vi "Write_mzMLFile.vi"(8 "error in (no error)":errorcluster, 10 "Signal Segment":T1={"SampleRate"=-1.0, "TrigDelay"=0.0, "SpecLength"=0.0, "DAQ_Range"=0.0, "Average#"=0, "Position"=[], "Spectrum"=[], "Calibr."=[], "Pressure"=-1.0, "Desp_LaserEnergy"=-1.0, "PI_LaserEnergy"=-1.0, "Voltages Table"=[], "ProcMode"=enum."None", "Threshold"=-1.0, "Comment"="", "TickCount"=0.0, "Time Stamp"=timestamp(0 s since 1904-01-01)} {"TickCount" format="%#.2f"}, 11 "Filename":path) -> (0 "error out":errorcluster)   [LabVIEW 2013]
uses:
  Signal_Segment.ctl
  ControlDef/ProcessingMode.ctl
panel:
  out "Sample Rate":dbl=100000000.0
  out "Depth":dbl=16384.0
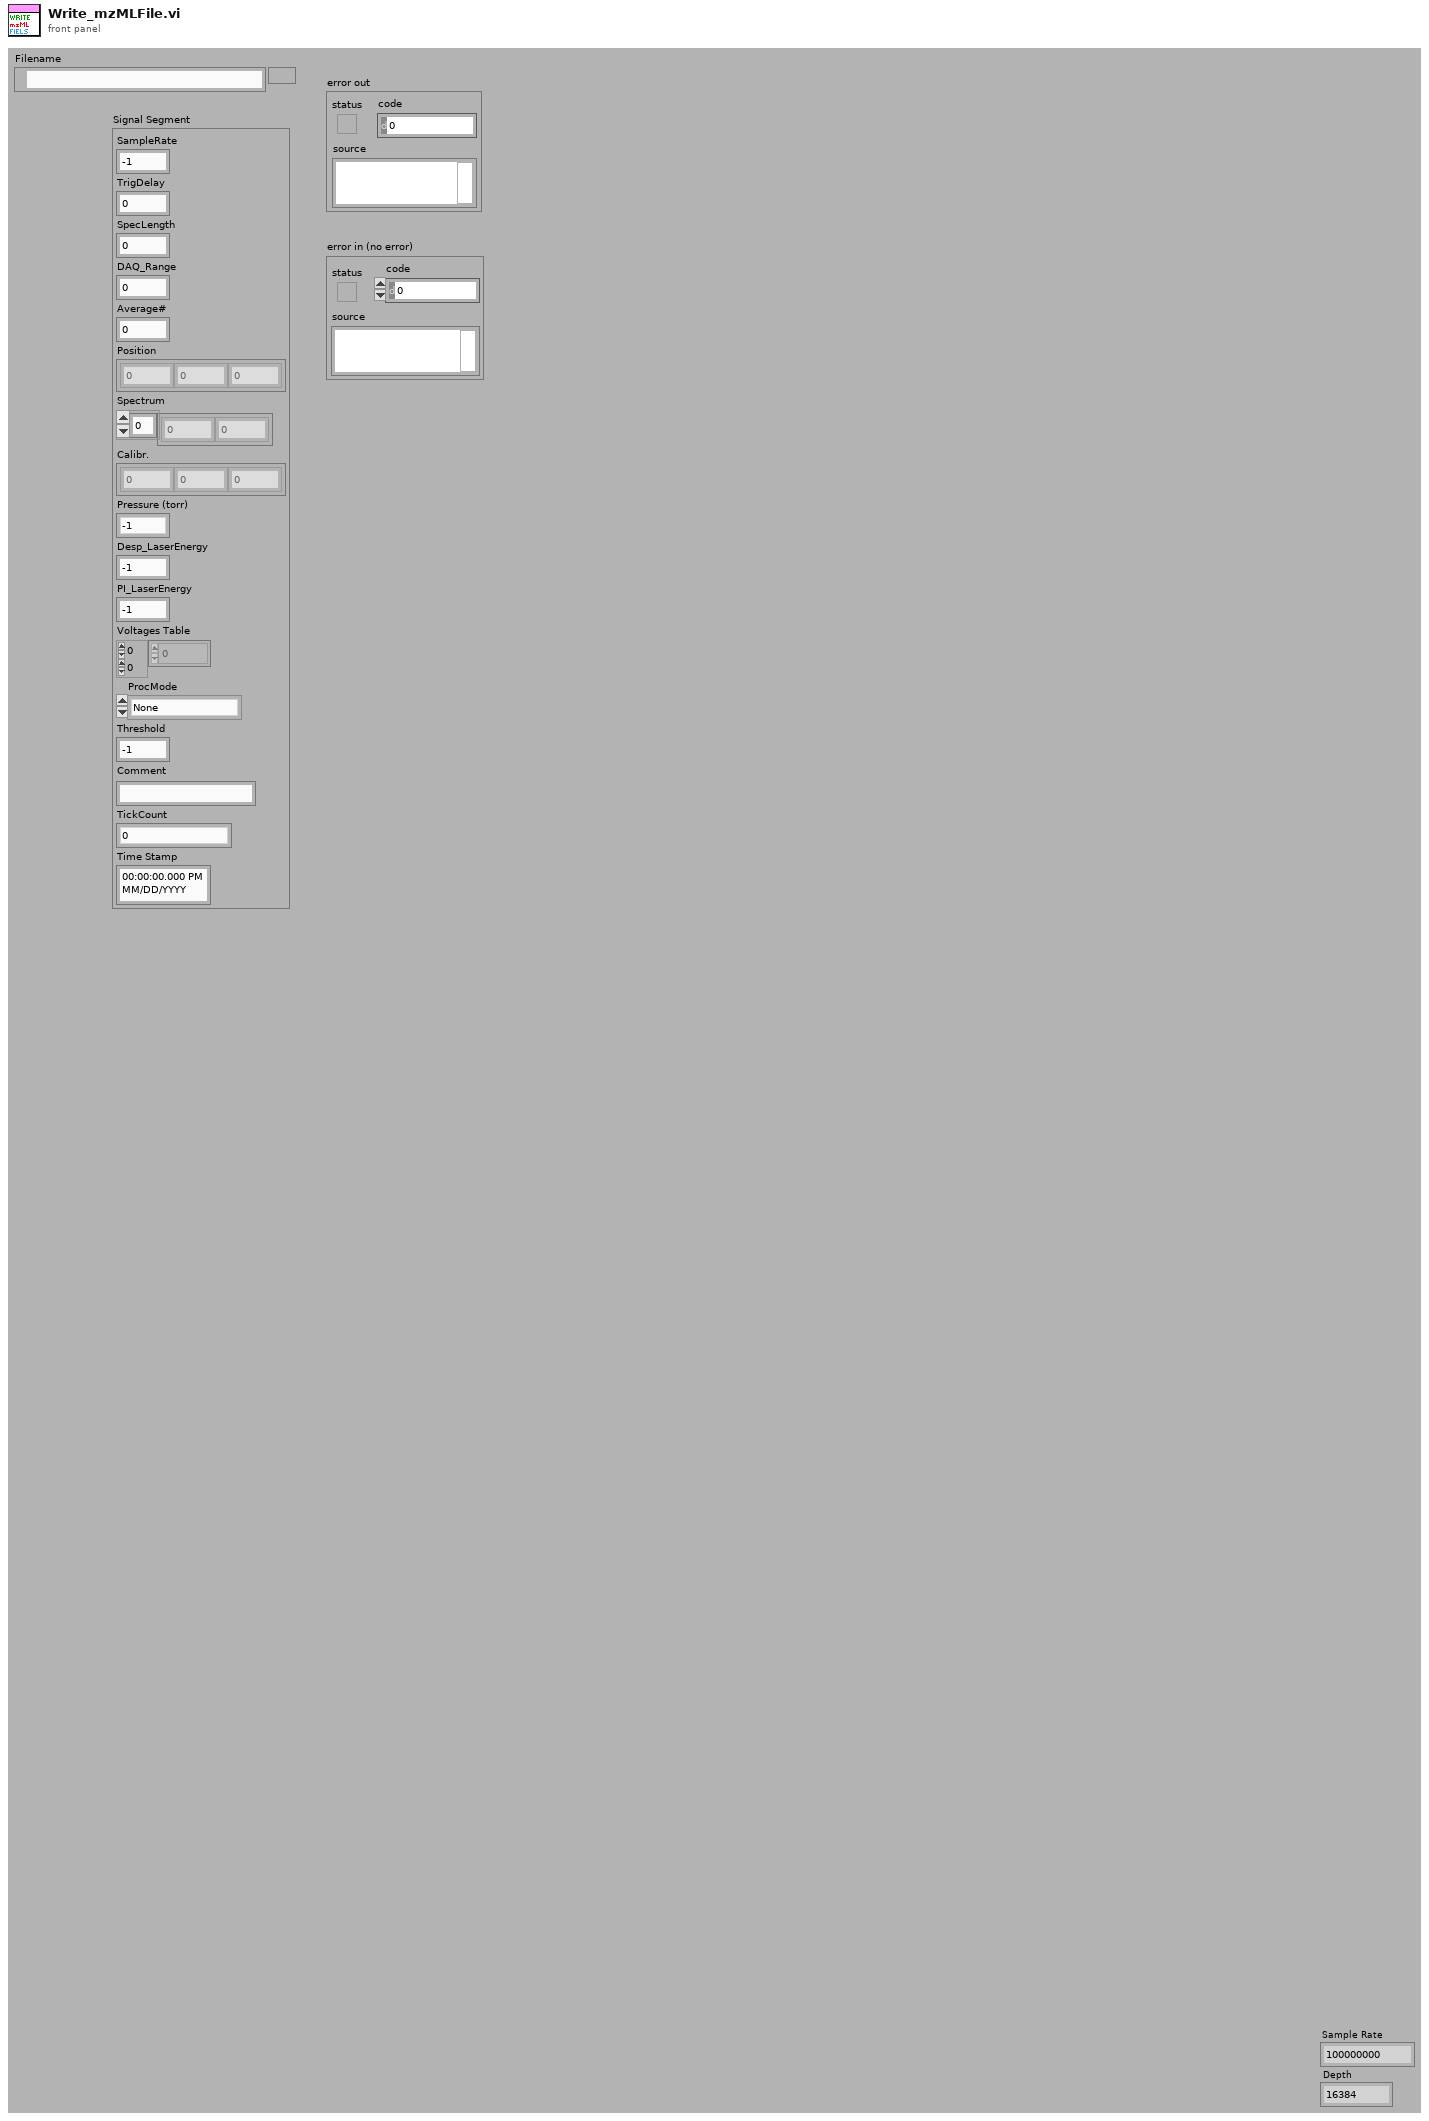
[diagram p1: front panel]
types:
  T1 = typedef "Signal_Segment.ctl" = cluster{"SampleRate":dbl, "TrigDelay":dbl, "SpecLength":dbl, "DAQ_Range":dbl, "Average#":i32, "Position":dbl[], "Spectrum":sgl[], "Calibr.":dbl[], "Pressure":dbl, "Desp_LaserEnergy":dbl, "PI_LaserEnergy":dbl, "Voltages Table":sgl[][], "ProcMode":T2, "Threshold":dbl, "Comment":string, "TickCount":dbl, "Time Stamp":timestamp}
  T2 = typedef "ProcessingMode.ctl" = enum16{"None", "Drop by Threshold", "TDC Simulate", "SetFilter"}
  T3 = enum16{"open", "replace", "create", "open or create", "replace or create", "replace or create with confirmation"}
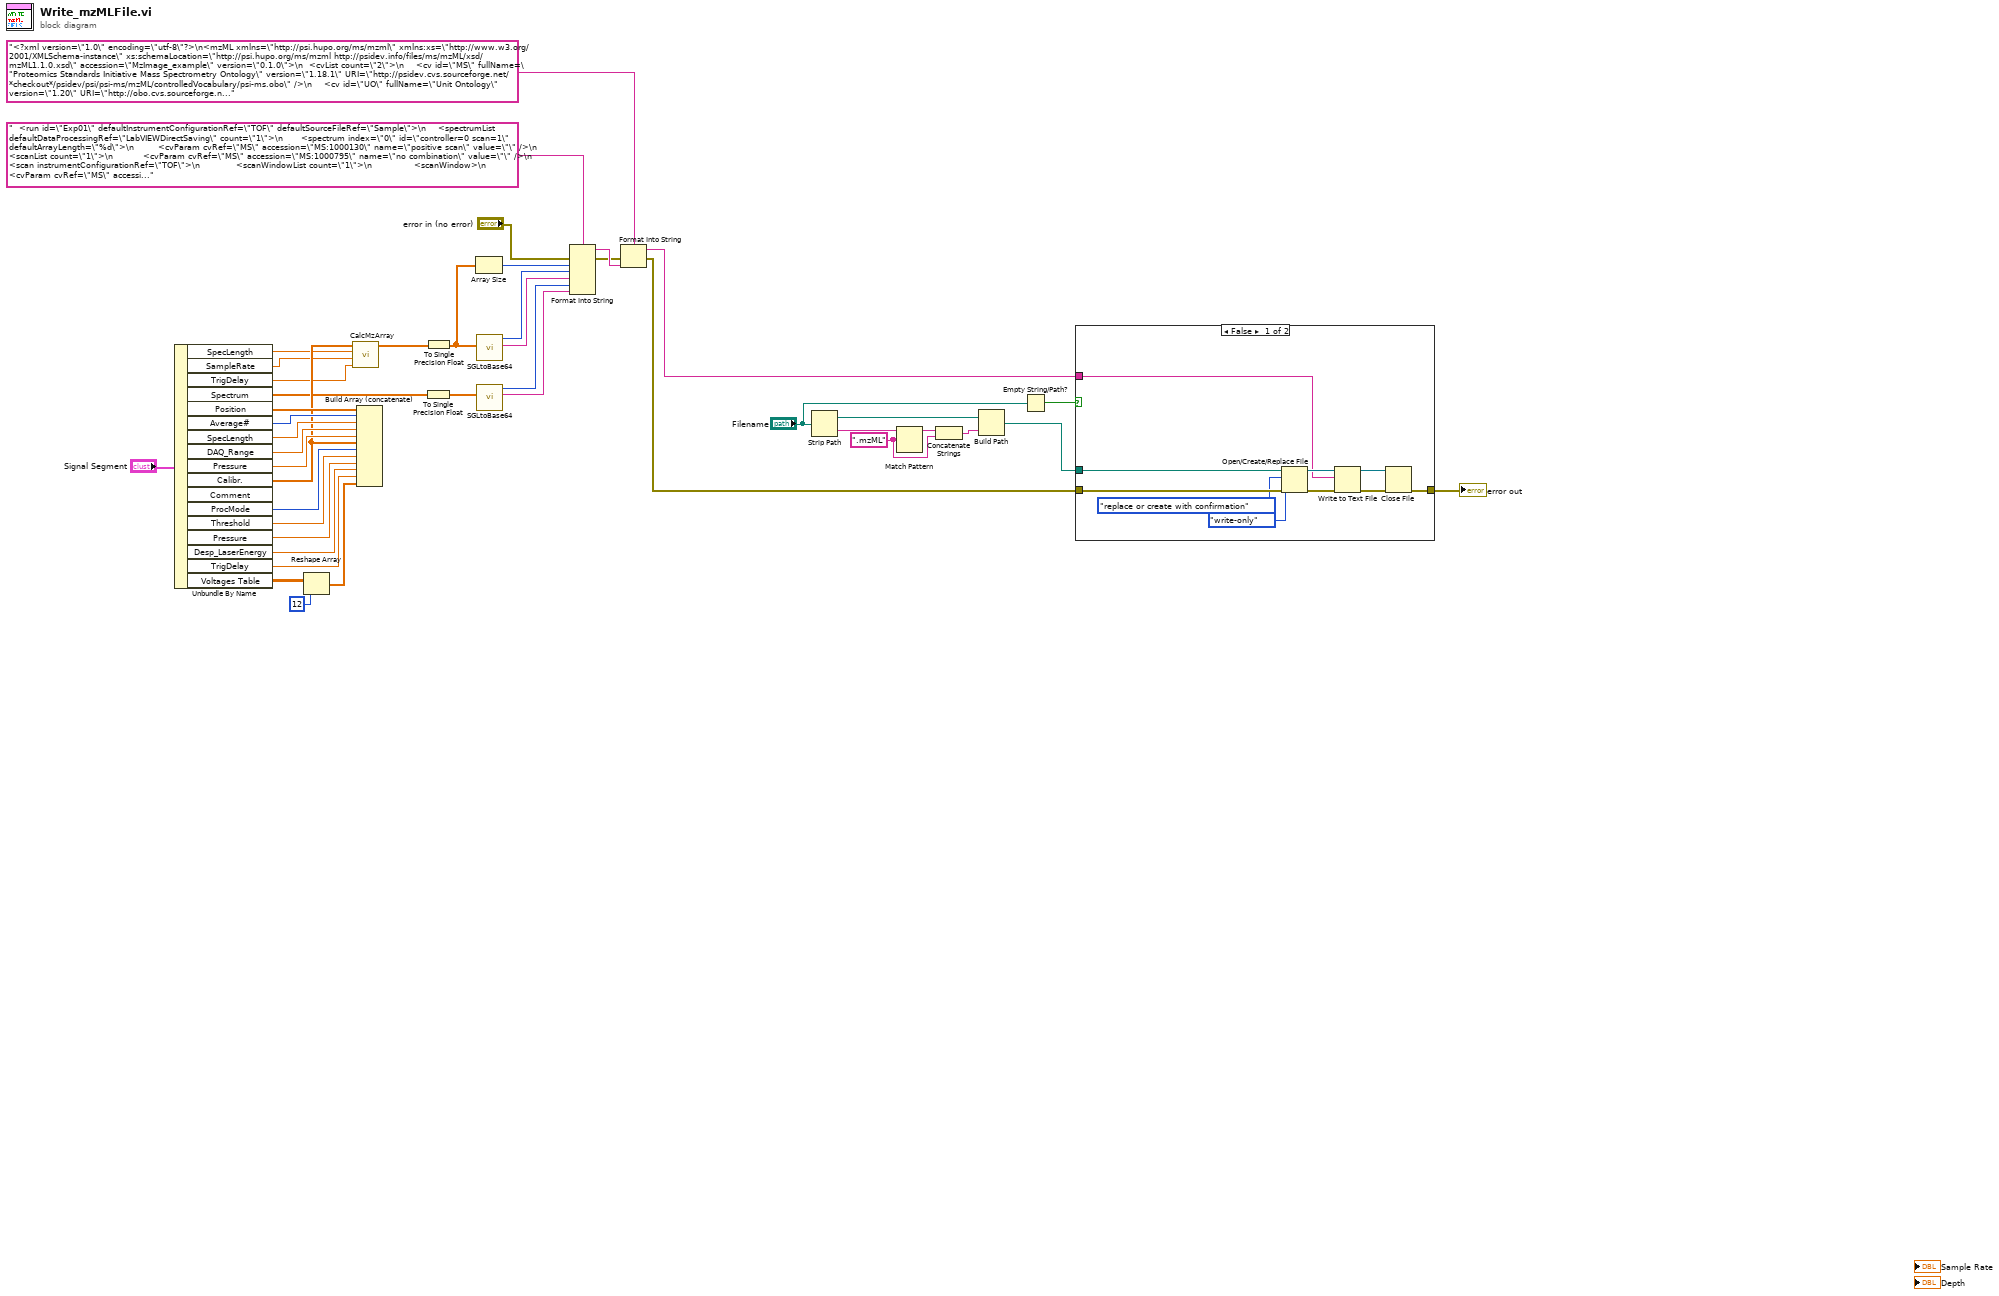
[diagram p0: block diagram]
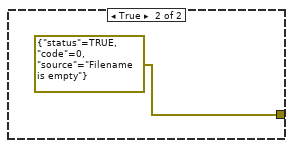
[diagram p2: hidden frame]
diagram:
  w30 = ".mzML" ("regular expression")
  n1 = Unbundle By Name("Signal Segment") -> ("SpecLength"=w2:dbl, "SampleRate"=w1:dbl, "TrigDelay"=w3:dbl, "Spectrum"=w4:sgl[], "Position"=w40:dbl[], "Average#"=w41:i32, "SpecLength"=w38:dbl, "DAQ_Range"=w42:dbl, "Pressure"=w37:dbl, "Calibr."=w21:dbl[], "ProcMode"=w36:T2, "Threshold"=w35:dbl, "Pressure"=w29:dbl, "Desp_LaserEnergy"=w28:dbl, "TrigDelay"=w22:dbl, "Voltages Table"=w24:sgl[][])  [unwired: 1 out]
  n2 = Reshape Array(w24, 12 ("dimension size")) -> (w23:sgl[])
  n3 = call "CalcMzArray.vi"("TrigDelay"=w3, "Sample Rate"=w1, "Depth"=w2, "mzCali. (a/b/c)"=w21) -> ("mzArray"=w5:dbl[])  [unwired: 7 in]
  n4 = Build Array (concatenate)(w40, w41, w38, w42, w37, w21, w36, w35, w29, w28, w22, w23) -> ()  [unwired: 1 out]
  n5 = To Single Precision Float(number=w4) -> (single precision float=w6:sgl[])
  n6 = To Single Precision Float(number=w5) -> (single precision float=w12:sgl[])
  n7 = Array Size(array=w12) -> (size(s)=w11:i32)
  n8 = call "SGLtoBase64.vi"("SGL Array"=w12) -> ("Base64 String"=w16:string, "length"=w15:i32)  [unwired: 9 in]
  n9 = call "SGLtoBase64.vi"("SGL Array"=w6) -> ("Base64 String"=w13:string, "length"=w14:i32)  [unwired: 9 in]
  n10 = Format Into String(format string="  <run id=\"Exp01\" defaultInstrumentConfigurationRef=\"TOF\" defaultSourceFileRef=\"Sample\">\n    <spectrumList defaultDataProcessingRef=\"LabVIEWDirectSaving\" count=\"1\">\n      <spectrum index=\"0\" id=\"controller=0 scan=1\" defaultArrayLength=\"%d\">\n        <cvParam cvRef=\"MS\" accession=\"MS:1000130\" name=\"positive scan\" value=\"\" />\n        <scanList count=\"1\">\n          <cvParam cvRef=\"MS\" accession=\"MS:1000795\" name=\"no combination\" value=\"\" />\n          <scan instrumentConfigurationRef=\"TOF\">\n            <scanWindowList count=\"1\">\n              <scanWindow>\n                <cvParam cvRef=\"MS\" accession=\"MS:1000501\" name=\"scan window lower limit\" value=\"0\" unitCvRef=\"MS\" unitAccession=\"MS:1000040\" unitName=\"m/z\" />\n                <cvParam cvRef=\"MS\" accession=\"MS:1000500\" name=\"scan window upper limit\" value=\"5000\" unitCvRef=\"MS\" unitAccession=\"MS:1000040\" unitName=\"m/z\" />\n              </scanWindow>\n            </scanWindowList>\n          </scan>\n        </scanList>\n        <binaryDataArrayList count=\"2\">\n          <binaryDataArray encodedLength=\"%d\">\n            <cvParam cvRef=\"MS\" accession=\"MS:1000514\" name=\"m/z array\" unitCvRef=\"MS\" unitAccession=\"MS:1000040\" unitName=\"m/z\" />\n            <cvParam cvRef=\"MS\" accession=\"MS:1000576\" name=\"no compression\" />\n            <cvParam cvRef=\"MS\" accession=\"MS:1000521\" name=\"32-bit float\" />\n            <binary>%s</binary>\n          </binaryDataArray>\n          <binaryDataArray encodedLength=\"%d\">\n            <cvParam cvRef=\"MS\" accession=\"MS:1000515\" name=\"intensity array\" unitCvRef=\"MS\" unitAccession=\"MS:1000131\" unitName=\"number of counts\" />\n            <cvParam cvRef=\"MS\" accession=\"MS:1000574\" name=\"zlib compression\" />\n            <cvParam cvRef=\"MS\" accession=\"MS:1000521\" name=\"32-bit float\" />\n            <binary>%s</binary>\n          </binaryDataArray>\n        </binaryDataArrayList>\n      </spectrum>\n    </spectrumList>\n  </run>", error in="error in (no error)", w11, w15, w16, w14, w13) -> (resulting string=w17:string, error out=w9:errorcluster)  [unwired: 1 in]
  n11 = Format Into String(format string="<?xml version=\"1.0\" encoding=\"utf-8\"?>\n<mzML xmlns=\"http://psi.hupo.org/ms/mzml\" xmlns:xs=\"http://www.w3.org/2001/XMLSchema-instance\" xs:schemaLocation=\"http://psi.hupo.org/ms/mzml http://psidev.info/files/ms/mzML/xsd/mzML1.1.0.xsd\" accession=\"MzImage_example\" version=\"0.1.0\">\n  <cvList count=\"2\">\n    <cv id=\"MS\" fullName=\"Proteomics Standards Initiative Mass Spectrometry Ontology\" version=\"1.18.1\" URI=\"http://psidev.cvs.sourceforge.net/*checkout*/psidev/psi/psi-ms/mzML/controlledVocabulary/psi-ms.obo\" />\n    <cv id=\"UO\" fullName=\"Unit Ontology\" version=\"1.20\" URI=\"http://obo.cvs.sourceforge.net/*checkout*/obo/obo/ontology/phenotype/unit.obo\" />\n  </cvList>\n  <fileDescription>\n    <fileContent>\n      <cvParam cvRef=\"MS\" accession=\"MS:1000442\" name=\"spectrum\" />\n    </fileContent>\n    <sourceFileList count=\"2\">\n      <sourceFile id=\"Sample\" name=\"\" location=\"\"></sourceFile>\n    </sourceFileList>\n  </fileDescription>\n  <softwareList count=\"1\">\n    <software id=\"software\" version=\"3.5\">\n      <cvParam cvRef=\"MS\" accession=\"MS:1000531\" name=\"software\" value=\"\" />\n    </software>\n  </softwareList>\n  <instrumentConfigurationList count=\"1\">\n    <instrumentConfiguration id=\"TOF\">\n      <cvParam cvRef=\"MS\" accession=\"MS:1000287\" name=\"time-of-flight mass spectrometer\" value=\"\" />\n      <componentList count=\"3\">\n        <source order=\"1\">\n          <cvParam cvRef=\"MS\" accession=\"MS:1000393\" name=\"laser desorption ionization\"></cvParam>\n        </source>\n        <analyzer order=\"2\">\n          <cvParam cvRef=\"MS\" accession=\"MS:1000084\" name=\"TOF\" value=\"\" />\n        </analyzer>\n        <detector order=\"3\">\n          <cvParam cvRef=\"MS\" accession=\"MS:1000114\" name=\"microchannel plate detector\" value=\"\" />\n        </detector>\n      </componentList>\n      <softwareRef ref=\"software\" />\n    </instrumentConfiguration>\n  </instrumentConfigurationList>\n  <dataProcessingList count=\"1\">\n    <dataProcessing id=\"LabVIEWDirectSaving\">\n      <processingMethod softwareRef=\"software\" order=\"1\">\n        <cvParam cvRef=\"MS\" accession=\"MS:1000544\" name=\"Conversion to mzML\" />\n      </processingMethod>\n    </dataProcessing>\n  </dataProcessingList>\n%s\n</mzML>", error in=w9, w17) -> (resulting string=w10:string, error out=w8:errorcluster)  [unwired: 1 in]
  n12 = Strip Path(path="Filename") -> (stripped path=w34:path, name=w33:string)
  n13 = Match Pattern(string=w33, regular expression=w30) -> (before substring=w31:string)  [unwired: 1 in, 3 out]
  n14 = Concatenate Strings(w31, w30) -> (w32:string)
  n15 = Build Path(base path=w34, name or relative path=w32) -> (appended path=w26:path)
  n16 = Empty String/Path?(string/path="Filename") -> (empty?=w27:bool)
  n17 = case shown="False" w27 {
    tunnel: w26 -> [w49 _]
    tunnel: w8 -> [w53 _]
    tunnel: [w47 errorcluster {"status"=TRUE, "code"=0, "source"="Filename is empty"} ("error out")] -> w20
    tunnel: w10 -> [w48 _]
    frame False {
      n18 = Open/Create/Replace File(file path (use dialog)=w49, error in=w53, operation (0:open)=T3."replace or create with confirmation", access (0:read/write)=enum16{"read/write", "read-only", "write-only"}."write-only") -> (refnum out=w50:refnum<file>, error out=w52:errorcluster)  [unwired: 2 in, 1 out]
      n19 = Write to Text File(file (use dialog)=w50, text=w48, error in=w52) -> (refnum out=w46:refnum<file>, error out=w51:errorcluster)  [unwired: 1 in, 1 out]
      n20 = Close File(refnum=w46, error in=w51) -> (error out=w47:errorcluster)  [unwired: 1 out]
    }
    frame True {
    }
  }
  "error out" <- w20
